vi "Host_Project 1.vi"() -> ()   [LabVIEW 2018]
uses:
  <vilib>/Instr/_visa.llb/VISA Configure Serial Port (Instr).vi
panel:
  in  "Стоп":bool
  out "Response":string
  in  "Отправка":bool
  in  "Request":string="led_on"
  in  "VISA resource name":refnum<visa-resource-name>
  # "Зажигание светодиода\nled_on\nled_off\n\nПроверка пинов\nD2_on\nD2_off\nD3_on\nD3_off\nD4_on\nD4_off\nD5_on\nD5_off"
  # "D6_on\nD6_off\nD7_on\nD7_off\nD8_on\nD8_off\nD9_on\nD9_off\nD10_on\nD10_off\nD11_on\nD11_off\nD12_on\nD12_off"
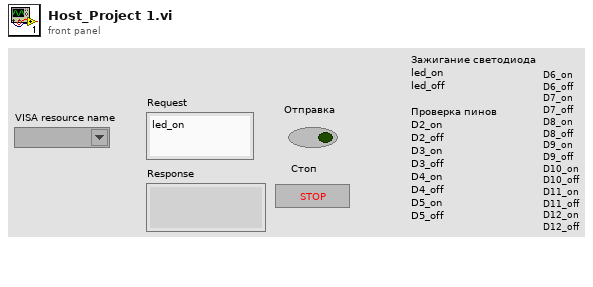
[diagram p1: front panel]
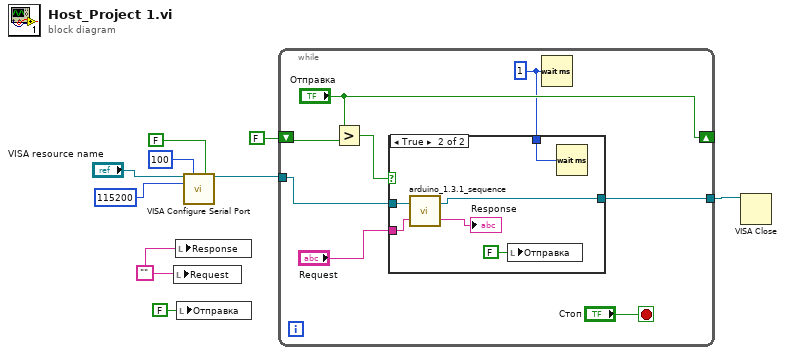
[diagram p0: block diagram]
diagram:
  w6 = ""
  n1 = local write "Request"(w6) -> ()
  n2 = local write "Response"(w6) -> ()
  n3 = local write "Отправка"(FALSE ("Отправка")) -> ()
  n4 = call-poly "VISA Configure Serial Port"("VISA resource name"="VISA resource name", "timeout (10sec)"=u32 100, "Enable Termination\nChar (T)"=FALSE ("Enable Termination\nChar (T)"), "baud rate (9600)"=u32 115200) -> ("VISA resource name out"=w1:refnum<visa-resource-name>)  [unwired: 10 in, 1 out]
  n5 = while {
    tunnel: w1 -> [w17]
    shift-right: ["Отправка"] -> _
    shift-left: FALSE -> [w16]
    tunnel: [w10] -> w7
    stop <- "Стоп" stop-if-true
    w12 = u32 1 ("milliseconds to wait")
    n6 = Greater?(x="Отправка", y=w16) -> (0:w14:bool)
    n7 = case shown="True" w14 {
      tunnel: w17 -> [w18 w22]
      tunnel: "Request" -> [_ w21]
      tunnel: w12 -> [_ w23]
      tunnel: [w18 w19] -> w10
      frame False {
      }
      frame True {
        n8 = call "arduino_1.3.1_sequence.vi"("Command 2"=w21, "VISA resource name 2"=w22) -> ("Commentary 2"=→"Response":string, "VISA resource name out"=w19:refnum<visa-resource-name>)
        n9 = local write "Отправка"(FALSE ("Отправка")) -> ()
        n10 = Wait (ms)(milliseconds to wait=w23) -> ()  [unwired: 1 out]
      }
    }
    n11 = Wait (ms)(milliseconds to wait=w12) -> ()  [unwired: 1 out]
  }
  n12 = VISA Close(VISA resource name=w7) -> ()  [unwired: 1 in, 1 out]
